vi "Добавить мишень (Sub VI).vi"(8 "error in":errorcluster) -> (0 "error out":errorcluster, 1 "отменен?":bool, 2 "Название мишени":string)   [LabVIEW 2013]
doc: "Ввод имени для новой мишени"
panel:
  in  "Введите название мишени":string
  in  "Отмена":bool
  in  "Сохранить настройки":bool
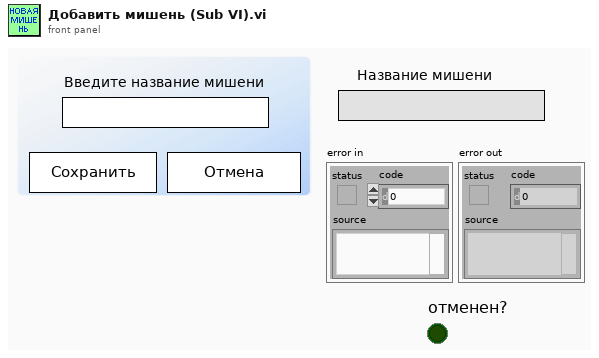
[diagram p1: front panel]
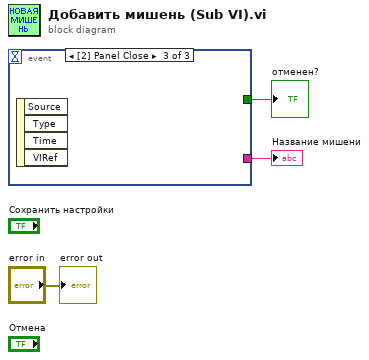
[diagram p0: block diagram]
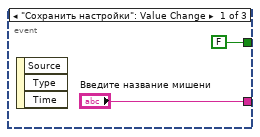
[diagram p2: hidden frame]
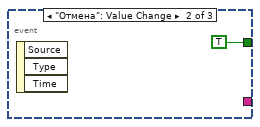
[diagram p3: hidden frame]
diagram:
  n1 = event shown="[2] Panel Close" {
    selector: _ -> [_ _ _]
    dyn-events: _ -> [_ _ _]
    timeout: _ -> [_ _ _]
    tunnel: ["Введите название мишени" _ _] -> w3
    tunnel: [FALSE ("Отмена") TRUE ("Отмена") _] -> w1
    event "Сохранить настройки": Value Change {
      n2 = event-data() -> ()  [unwired: 1 in, 3 out]
    }
    event "Отмена": Value Change {
      n3 = event-data() -> ()  [unwired: 1 in, 3 out]
    }
    event Panel Close {
      n4 = event-data() -> ()  [unwired: 1 in, 4 out]
    }
  }
  "Название мишени" <- w3
  "отменен?" <- w1
  "error out" <- "error in"
